vi "CRYTree Manuplate.vi"(4 "sData":string[](array[string]), 6 "Type":enum16{"Curves", "Values", "Results", "WFM"}(ring), 7 "sAction":string, 8 "sData Sub":string[](array[string]), 9 "nData":i32[](array[numeric]), 10 "sOption":string, 11 "Tree in":refnum<vi>) -> (0 "bResult Out":bool, 1 "sData Out":string[](array[string]), 2 "nData Out":i32[](array[numeric]), 3 "Tree Out":refnum<vi>)   [LabVIEW 2013]
uses:
  Global/CRYCurve Library Global.vi
panel:
  in  "Tags":string[](array[string])
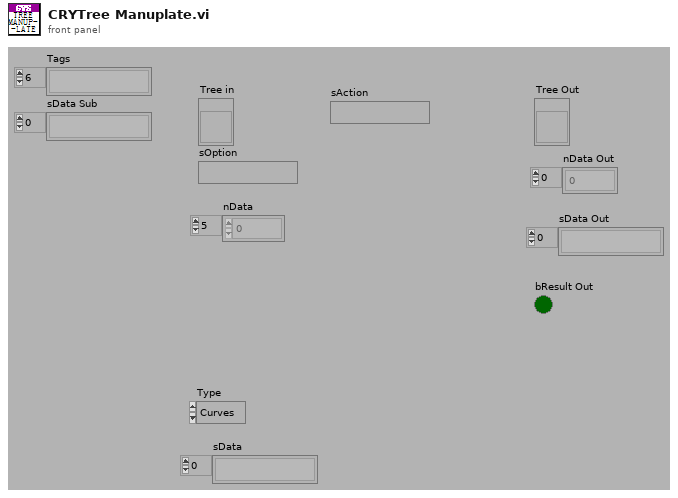
[diagram p1: front panel]
types:
  T1 = cluster{"Active Item Row Number":i32, "nData 2":i32}
  T2 = cluster{"Active Item Row Number":i32, "nData 2":i32}[]
  T3 = typedef "CRYCurveLib Info Cluster.ctl" = cluster{"GroupingState":string}
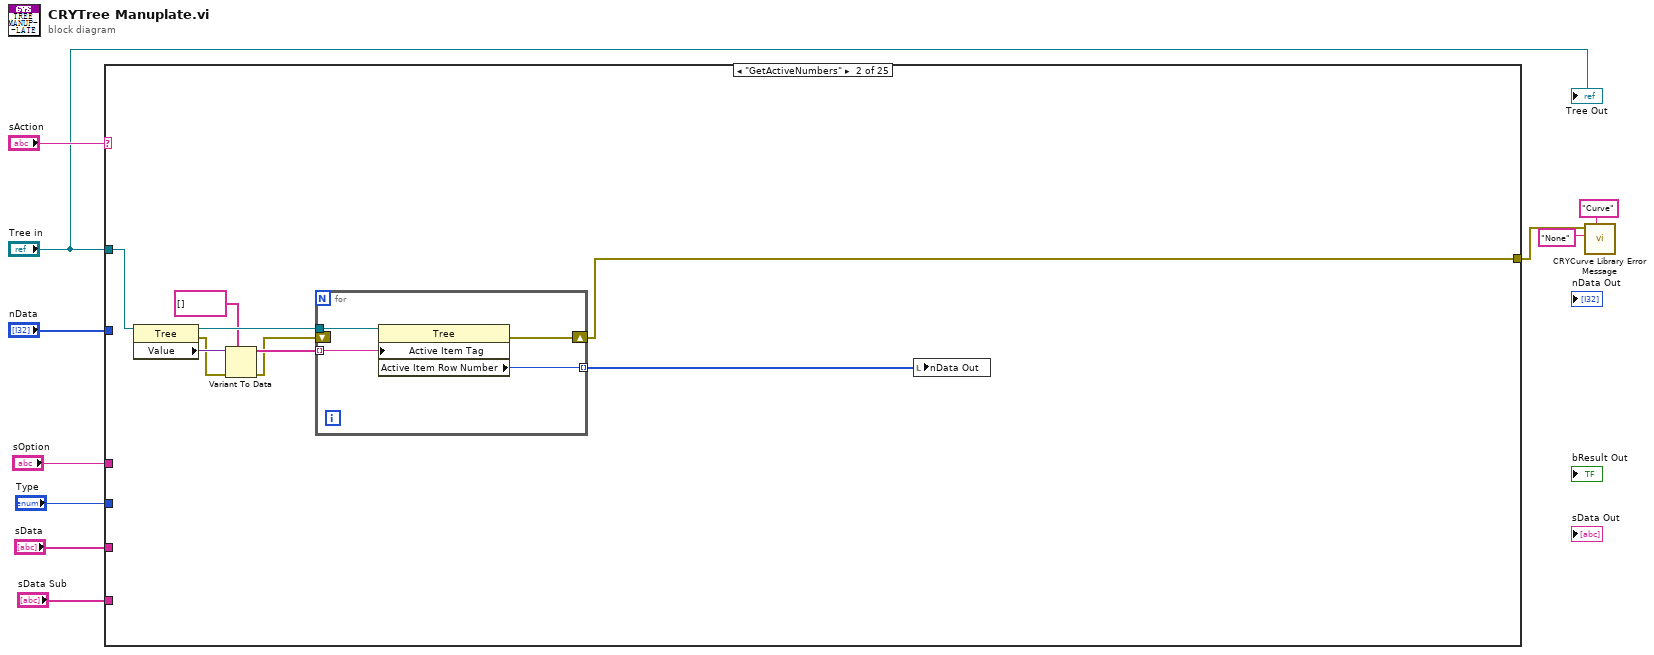
[diagram p0: block diagram]
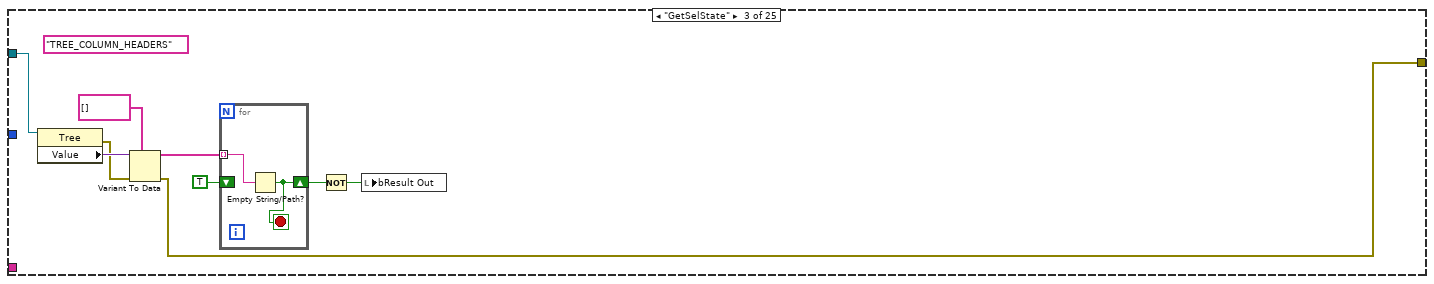
[diagram p3: hidden frame]
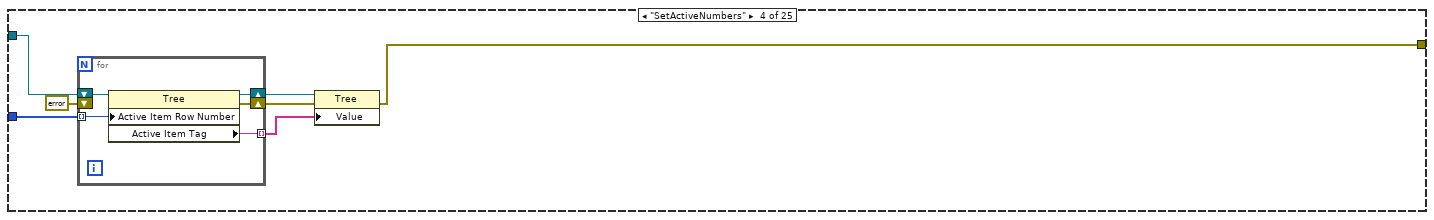
[diagram p4: hidden frame]
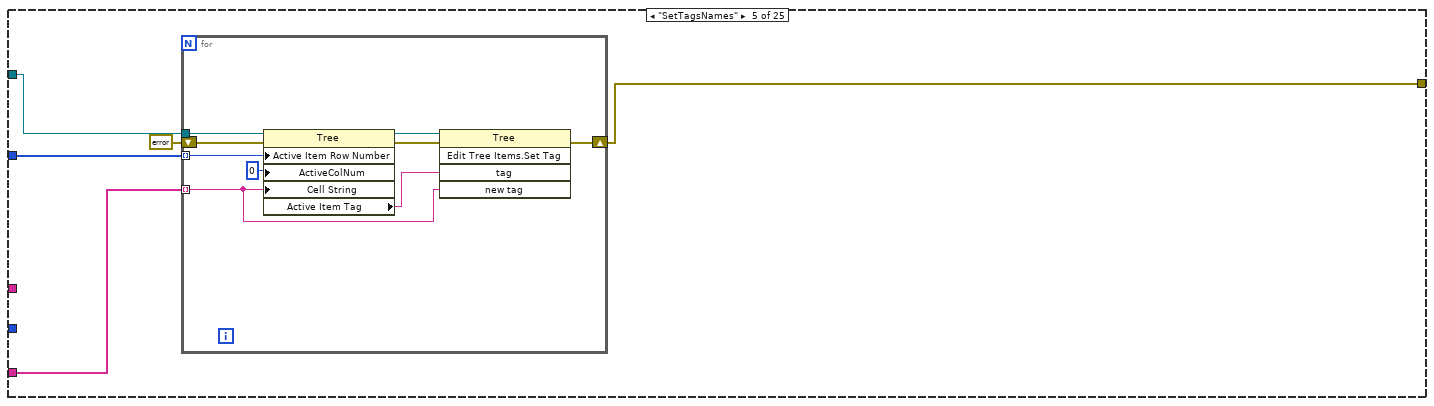
[diagram p5: hidden frame]
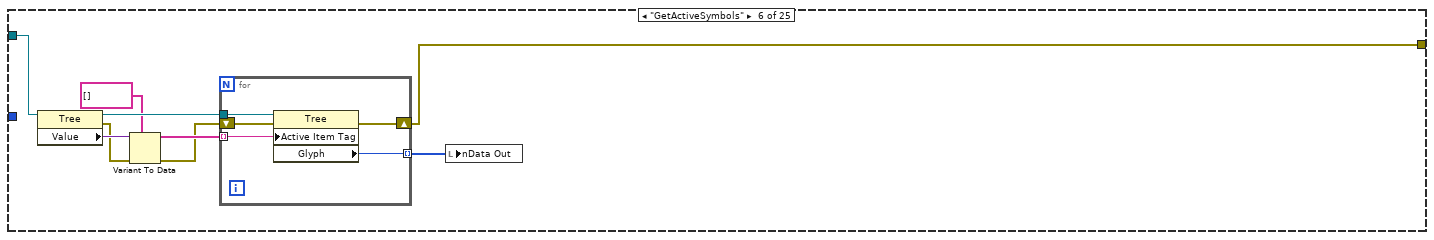
[diagram p6: hidden frame]
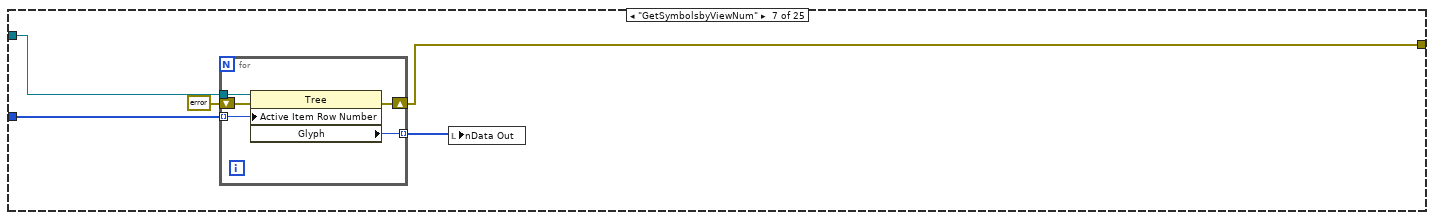
[diagram p7: hidden frame]
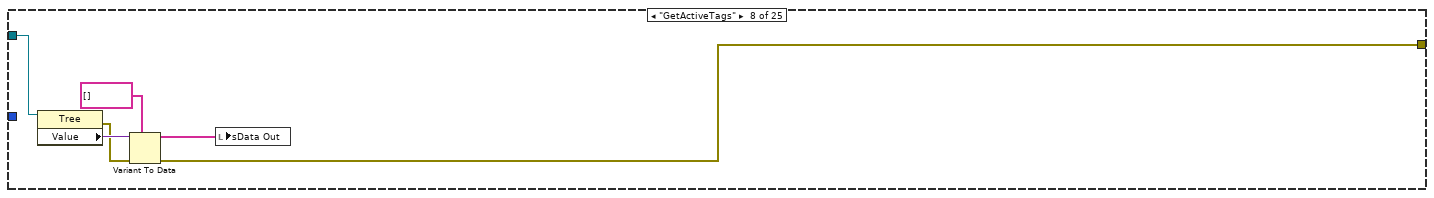
[diagram p8: hidden frame]
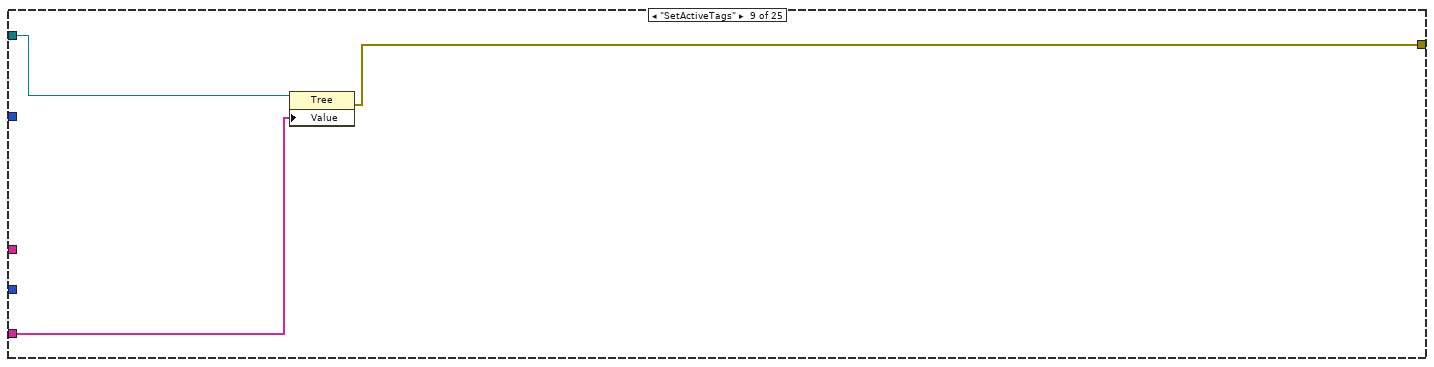
[diagram p9: hidden frame]
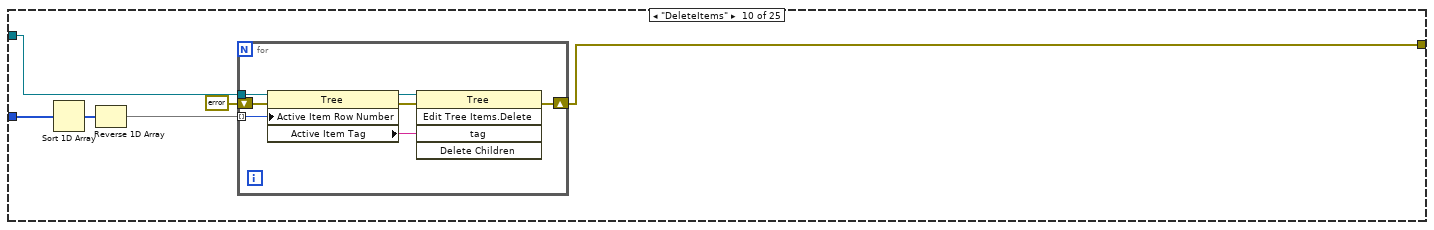
[diagram p10: hidden frame]
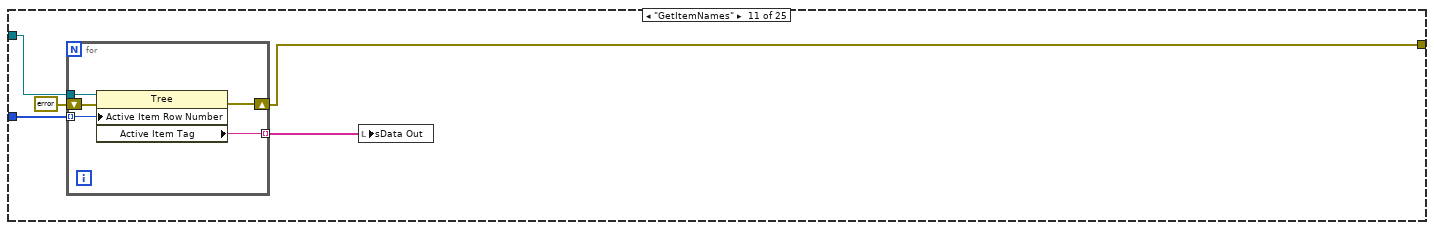
[diagram p11: hidden frame]
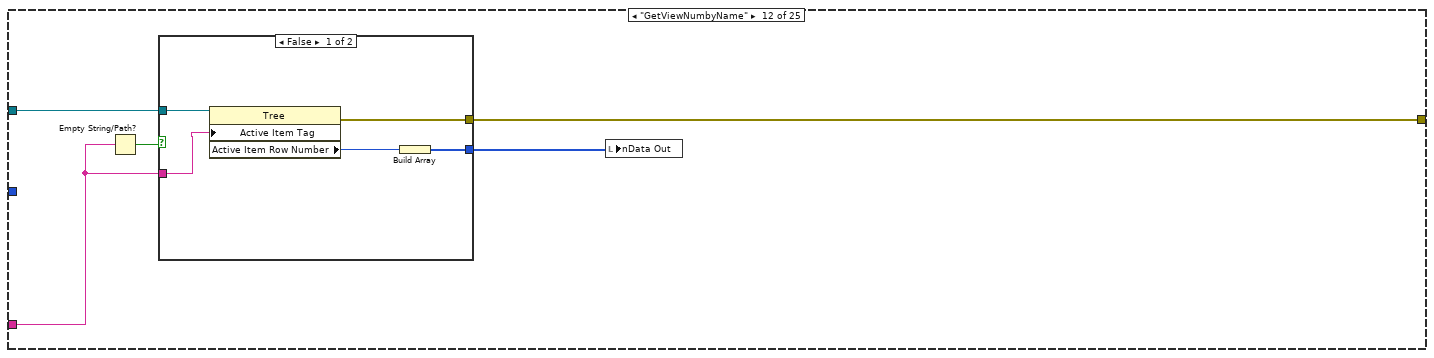
[diagram p12: hidden frame]
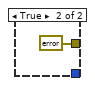
[diagram p13: hidden frame]
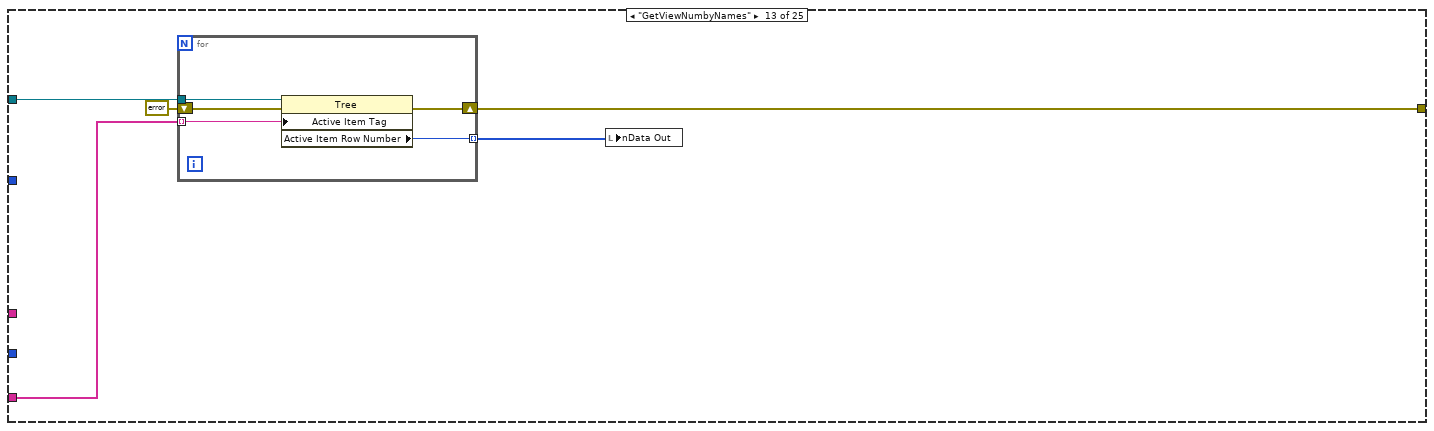
[diagram p14: hidden frame]
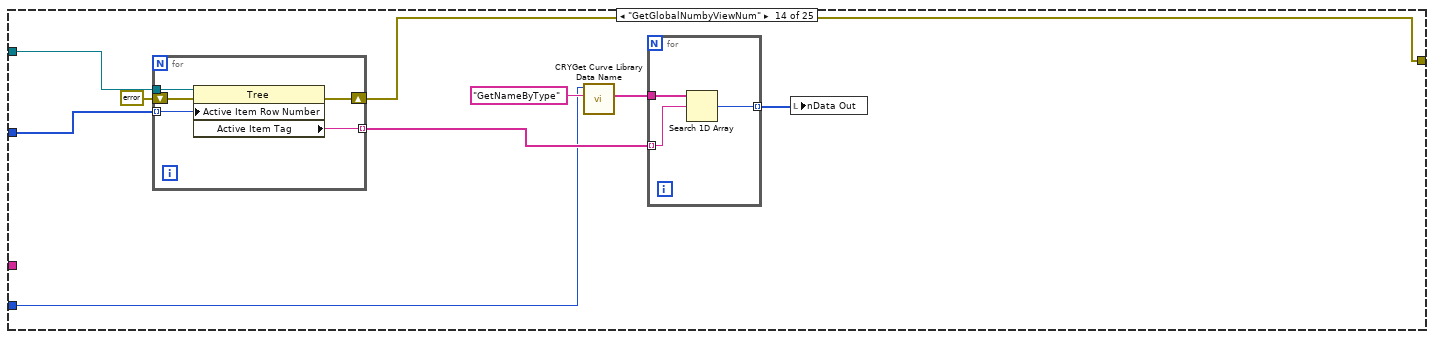
[diagram p15: hidden frame]
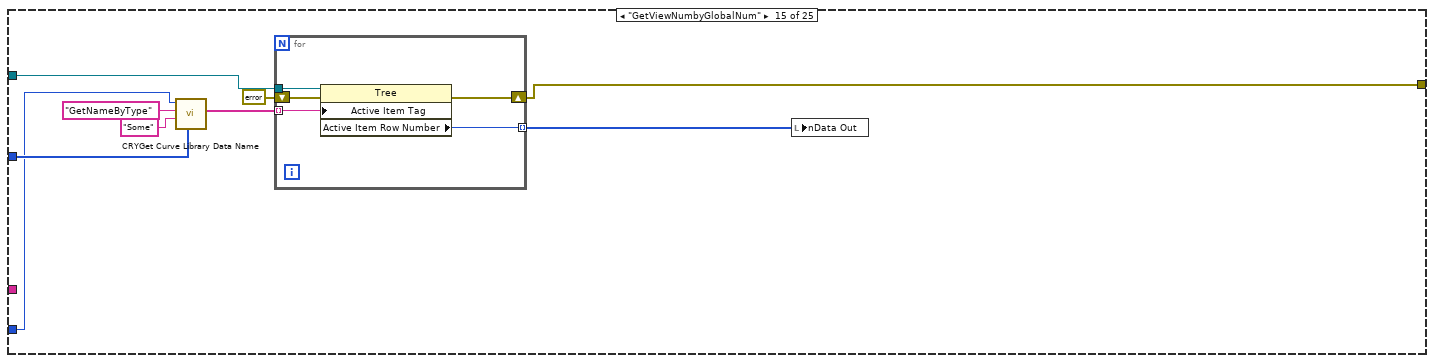
[diagram p16: hidden frame]
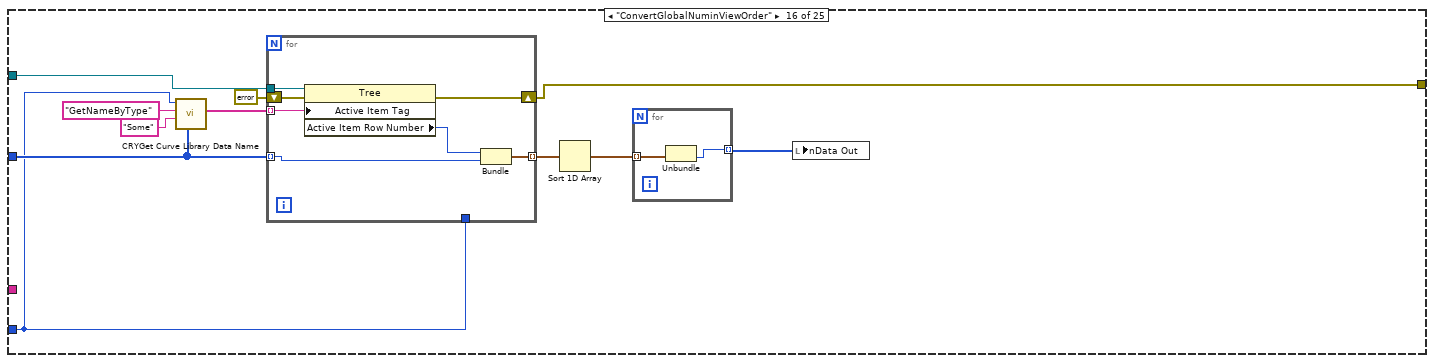
[diagram p17: hidden frame]
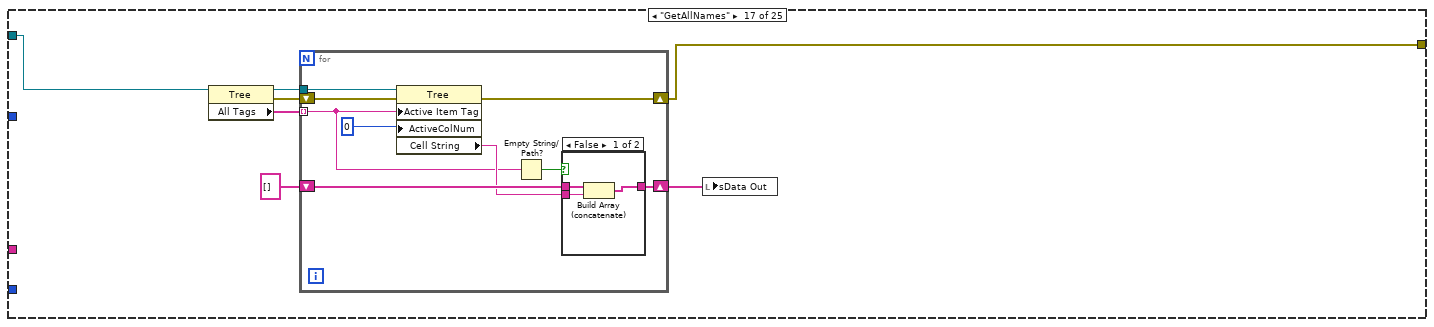
[diagram p18: hidden frame]
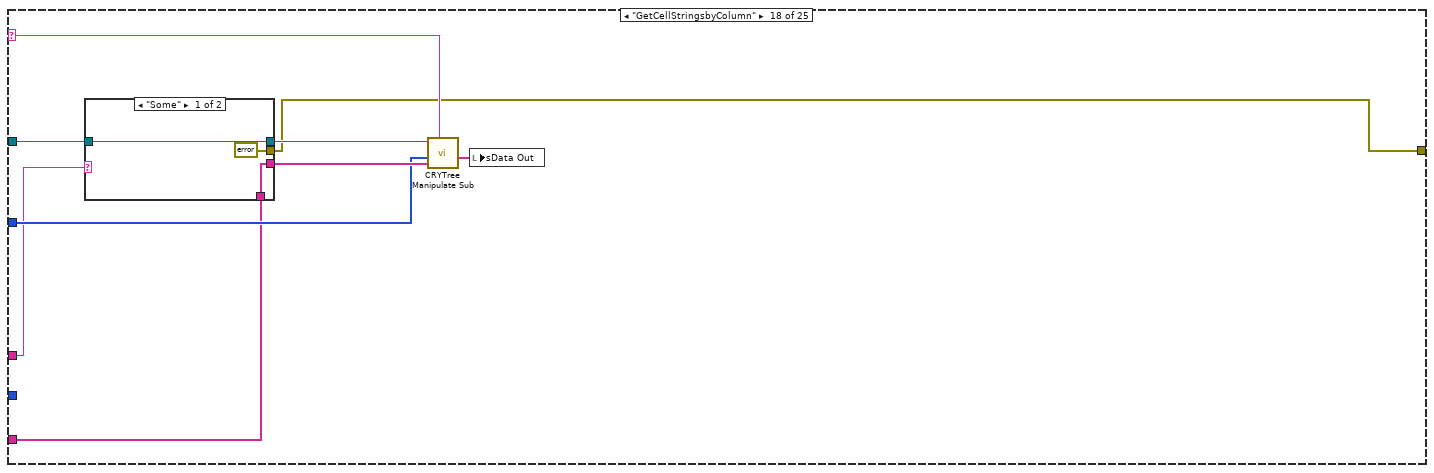
[diagram p20: hidden frame]
diagram:
  n1 = case shown="\"GetActiveNumbers\"" "sAction" {
    selector: "sAction" -> [_ _ _ _ _ _ _ _ _ _ _ _ _ _ _ _ _ w212 _ _ _ _ _ _ _]
    tunnel: "Tree in" -> [_ w16 w30 w41 w51 w65 w77 w88 w93 w99 w111 w121 w132 w146 w163 w176 w193 w214 w229 w245 w257 w327 w372 w735 w761]
    tunnel: "nData" -> [_ _ _ w39 w50 _ w78 _ _ w97 w110 _ _ w145 w160 w172 _ w216 _ _ w256 _ w373 w732 w763]
    tunnel: "sOption" -> [_ _ _ _ _ _ _ _ _ _ _ w118 _ _ _ _ _ w211 _ _ w252 _ w369 _ _]
    tunnel: "Type" -> [_ _ _ _ _ _ _ _ _ _ _ _ _ w140 w157 w171 _ _ _ _ _ _ _ _ _]
    tunnel: "sData" -> [_ _ _ _ w49 _ _ _ w92 _ _ _ w130 _ _ _ _ w210 _ _ _ w325 w368 _ w760]
    tunnel: "sData Sub" -> [_ _ _ _ _ _ _ _ _ _ _ _ _ _ _ _ _ _ _ _ _ _ _ _ _]
    tunnel: [_ w13 w24 w35 w48 w61 w75 w85 w91 w95 w108 w117 w128 w139 w156 w170 w189 w209 w226 w244 w251 w323 w367 w726 w759] -> w1
    frame Default {
    }
    frame "GetActiveNumbers" {
      n2 = property class="Tree"(reference=w16) -> (reference out=w17:refnum<vi>, error out=w12:errorcluster, "Value"=w19:variant)  [unwired: 1 in]
      n3 = Variant To Data(error in=w12, type=string[] [] ("Value"), Variant=w19) -> (data=w18:string[], error out=w11:errorcluster)
      n4 = for {
        tunnel: w17 -> [w23]
        tunnel: w18 -> [w21] mode=indexing
        tunnel: [w22] -> w15 mode=indexing
        shift-right: [w20] -> w13
        shift-left: w11 -> [_]
        n5 = property class="Tree"(reference=w23, "Active Item Tag"=w21) -> (error out=w20:errorcluster, "Active Item Row Number"=w22:i32)  [unwired: 1 in, 1 out]
      }
      n6 = local write "nData Out"(w15) -> ()
    }
    frame "GetSelState" {
      (unwired) "TREE_COLUMN_HEADERS" ("x")
      n7 = property class="Tree"(reference=w30) -> (error out=w25:errorcluster, "Value"=w32:variant)  [unwired: 1 in, 1 out]
      n8 = Variant To Data(error in=w25, type=string[] [] ("Value"), Variant=w32) -> (data=w31:string[], error out=w24:errorcluster)
      n9 = for {
        tunnel: w31 -> [w34] mode=indexing
        shift-right: [w33] -> w27
        shift-left: TRUE -> [_]
        stop <- w33 stop-if-true
        n10 = Empty String/Path?(string/path=w34) -> (empty?=w33:bool)
      }
      n11 = Not(x=w27) -> (.not. x?=w26:bool)
      n12 = local write "bResult Out"(w26) -> ()
    }
    frame "SetActiveNumbers" {
      n13 = for {
        tunnel: [w45] -> w38 mode=indexing
        tunnel: w39 -> [w43] mode=indexing
        shift-right: [w44] -> w40
        shift-left: w41 -> [w46]
        shift-right: [w42] -> w37
        shift-left: errorcluster {"status"=FALSE, "code"=0, "source"=""} ("error out") -> [_]
        n14 = property class="Tree"(reference=w46, "Active Item Row Number"=w43) -> (reference out=w44:refnum<vi>, error out=w42:errorcluster, "Active Item Tag"=w45:string)  [unwired: 1 in]
      }
      n15 = property class="Tree"(reference=w40, error in=w37, "Value"=w38) -> (error out=w35:errorcluster)  [unwired: 1 out]
    }
    frame "SetTagsNames" {
      n16 = for {
        tunnel: w50 -> [w60] mode=indexing
        tunnel: w51 -> [w58]
        tunnel: w49 -> [w56] mode=indexing
        shift-right: [w54] -> w48
        shift-left: errorcluster {"status"=FALSE, "code"=0, "source"=""} ("error out") -> [w53]
        n17 = property class="Tree"(reference=w58, error in=w53, "Active Item Row Number"=w60, "ActiveColNum"=0 ("Active Cell:Active Column Number"), "Cell String"=w56) -> (reference out=w57:refnum<vi>, error out=w52:errorcluster, "Active Item Tag"=w55:string)
        n18 = invoke class="Tree" method="Edit Tree Items.Set Tag"(reference=w57, error in=w52, "tag"=w55, "new tag"=w56) -> (error out=w54:errorcluster)  [unwired: 1 in, 4 out]
      }
    }
    frame "GetActiveSymbols" {
      n19 = property class="Tree"(reference=w65) -> (reference out=w67:refnum<vi>, error out=w63:errorcluster, "Value"=w69:variant)  [unwired: 1 in]
      n20 = Variant To Data(error in=w63, type=string[] [] ("Selected Rows"), Variant=w69) -> (data=w68:string[], error out=w62:errorcluster)
      n21 = for {
        tunnel: w67 -> [w74]
        tunnel: w68 -> [w72] mode=indexing
        tunnel: [w73] -> w64 mode=indexing
        shift-right: [w70] -> w61
        shift-left: w62 -> [w71]
        n22 = property class="Tree"(reference=w74, error in=w71, "Active Item Tag"=w72) -> (error out=w70:errorcluster, "Glyph"=w73:i32)  [unwired: 1 out]
      }
      n23 = local write "nData Out"(w64) -> ()
    }
    frame "GetSymbolsbyViewNum" {
      n24 = for {
        tunnel: w77 -> [w84]
        tunnel: w78 -> [w83] mode=indexing
        tunnel: [w82] -> w79 mode=indexing
        shift-right: [w81] -> w75
        shift-left: errorcluster {"status"=FALSE, "code"=0, "source"=""} ("error out") -> [w80]
        n25 = property class="Tree"(reference=w84, error in=w80, "Active Item Row Number"=w83) -> (error out=w81:errorcluster, "Glyph"=w82:i32)  [unwired: 1 out]
      }
      n26 = local write "nData Out"(w79) -> ()
    }
    frame "GetActiveTags" {
      n27 = property class="Tree"(reference=w88) -> (error out=w86:errorcluster, "Value"=w90:variant)  [unwired: 1 in, 1 out]
      n28 = Variant To Data(error in=w86, type=string[] [] ("Selected Rows"), Variant=w90) -> (data=w87:string[], error out=w85:errorcluster)
      n29 = local write "sData Out"(w87) -> ()
    }
    frame "SetActiveTags" {
      n30 = property class="Tree"(reference=w93, "Value"=w92) -> (error out=w91:errorcluster)  [unwired: 1 in, 1 out]
    }
    frame "DeleteItems" {
      n31 = Sort 1D Array(array=w97) -> (sorted array=w98:i32[])
      n32 = Reverse 1D Array(array=w98) -> (reversed array=w96:i32[])
      n33 = for {
        tunnel: w99 -> [w105]
        tunnel: w96 -> [w104] mode=indexing
        shift-right: [w101] -> w95
        shift-left: errorcluster {"status"=FALSE, "code"=0, "source"=""} ("error out") -> [w100]
        n34 = property on="Property Node" class="Tree"(reference=w105, error in=w100, "Active Item Row Number"=w104) -> (reference out=w103:refnum<vi>, error out=w102:errorcluster, "Active Item Tag"=w106:string)
        n35 = invoke class="Tree" method="Edit Tree Items.Delete"(reference=w103, error in=w102, "tag"=w106) -> (error out=w101:errorcluster)  [unwired: 2 in, 4 out]
      }
    }
    frame "GetItemNames" {
      n36 = for {
        tunnel: w111 -> [w116]
        tunnel: w110 -> [w115] mode=indexing
        tunnel: [w114] -> w109 mode=indexing
        shift-right: [w113] -> w108
        shift-left: errorcluster {"status"=FALSE, "code"=0, "source"=""} ("error out") -> [w112]
        n37 = property on="Property Node" class="Tree"(reference=w116, error in=w112, "Active Item Row Number"=w115) -> (error out=w113:errorcluster, "Active Item Tag"=w114:string)  [unwired: 1 out]
      }
      n38 = local write "sData Out"(w109) -> ()
    }
    frame "GetViewNumbyName" {
      n39 = Empty String/Path?(string/path=w118) -> (empty?=w119:bool)
      n40 = case shown="False" w119 {
        tunnel: w121 -> [w126 _]
        tunnel: [w124 _] -> w120
        tunnel: w118 -> [w123 _]
        tunnel: [w122 errorcluster {"status"=FALSE, "code"=0, "source"=""} ("error out")] -> w117
        frame False {
          n41 = property class="Tree"(reference=w126, "Active Item Tag"=w123) -> (error out=w122:errorcluster, "Active Item Row Number"=w125:i32)  [unwired: 1 in, 1 out]
          n42 = Build Array(w125) -> (w124:i32[])
        }
        frame True {
        }
      }
      n43 = local write "nData Out"(w120) -> ()
    }
    frame "GetViewNumbyNames" {
      n44 = for {
        tunnel: w132 -> [w137]
        tunnel: [w136] -> w131 mode=indexing
        tunnel: w130 -> [w135] mode=indexing
        shift-right: [w134] -> w128
        shift-left: errorcluster {"status"=FALSE, "code"=0, "source"=""} ("error out") -> [w133]
        n45 = property class="Tree"(reference=w137, error in=w133, "Active Item Tag"=w135) -> (error out=w134:errorcluster, "Active Item Row Number"=w136:i32)  [unwired: 1 out]
      }
      n46 = local write "nData Out"(w131) -> ()
    }
    frame "GetGlobalNumbyViewNum" {
      n47 = for {
        tunnel: w146 -> [w154]
        tunnel: w145 -> [w153] mode=indexing
        tunnel: [w152] -> w143 mode=indexing
        shift-right: [w151] -> w139
        shift-left: errorcluster {"status"=FALSE, "code"=0, "source"=""} ("error out") -> [w150]
        n48 = property on="Property Node" class="Tree"(reference=w154, error in=w150, "Active Item Row Number"=w153) -> (error out=w151:errorcluster, "Active Item Tag"=w152:string)  [unwired: 1 out]
      }
      n49 = call "CRYGet Curve Library Data Name.vi"("sAction"="GetNameByType", "Type"=w140) -> ("sNames"=w142:string[])  [unwired: 6 in, 3 out]
      n50 = for {
        tunnel: w143 -> [w148] mode=indexing
        tunnel: w142 -> [w149]
        tunnel: [w147] -> w141 mode=indexing
        n51 = Search 1D Array(1D array=w149, element=w148) -> (index of element=w147:i32)  [unwired: 1 in]
      }
      n52 = local write "nData Out"(w141) -> ()
    }
    frame "GetViewNumbyGlobalNum" {
      n53 = call "CRYGet Curve Library Data Name.vi"("nData"=w160, "sOption"="Some", "sAction"="GetNameByType", "Type"=w157) -> ("sNames"=w159:string[])  [unwired: 4 in, 3 out]
      n54 = for {
        tunnel: w163 -> [w168]
        tunnel: w159 -> [w166] mode=indexing
        tunnel: [w167] -> w158 mode=indexing
        shift-right: [w165] -> w156
        shift-left: errorcluster {"status"=FALSE, "code"=0, "source"=""} ("error out") -> [w164]
        n55 = property on="Property Node" class="Tree"(reference=w168, error in=w164, "Active Item Tag"=w166) -> (error out=w165:errorcluster, "Active Item Row Number"=w167:i32)  [unwired: 1 out]
      }
      n56 = local write "nData Out"(w158) -> ()
    }
    frame "ConvertGlobalNuminViewOrder" {
      n57 = call "CRYGet Curve Library Data Name.vi"("nData"=w172, "sOption"="Some", "sAction"="GetNameByType", "Type"=w171) -> ("sNames"=w177:string[])  [unwired: 4 in, 3 out]
      n58 = for {
        tunnel: w176 -> [w188]
        tunnel: w177 -> [w184] mode=indexing
        tunnel: [w186] -> w175 mode=indexing
        tunnel: w172 -> [w185] mode=indexing
        tunnel: w171 -> [_]
        shift-right: [w183] -> w170
        shift-left: errorcluster {"status"=FALSE, "code"=0, "source"=""} ("error out") -> [w182]
        n59 = property on="Property Node" class="Tree"(reference=w188, error in=w182, "Active Item Tag"=w184) -> (error out=w183:errorcluster, "Active Item Row Number"=w187:i32)  [unwired: 1 out]
        n60 = Bundle("Active Item Row Number"=w187, "nData 2"=w185) -> (w186:T1)  [unwired: 1 in]
      }
      n61 = Sort 1D Array(array=w175) -> (sorted array=w174:T2)
      n62 = for {
        tunnel: w174 -> [w181] mode=indexing
        tunnel: [w180] -> w173 mode=indexing
        n63 = Unbundle(w181) -> ("nData 2"=w180:i32)  [unwired: 1 out]
      }
      n64 = local write "nData Out"(w173) -> ()
    }
    frame "GetAllNames" {
      n65 = property class="Tree"(reference=w193) -> (reference out=w192:refnum<vi>, error out=w190:errorcluster, "All Tags"=w191:string[])  [unwired: 1 in]
      n66 = for {
        tunnel: w192 -> [w199]
        shift-right: [w202] -> w195
        shift-left: string[] [] -> [w203]
        tunnel: w191 -> [w198] mode=indexing
        shift-right: [w196] -> w189
        shift-left: w190 -> [w197]
        n67 = property class="Tree"(reference=w199, error in=w197, "Active Item Tag"=w198, "ActiveColNum"=0 ("Active Cell:Active Column Number")) -> (error out=w196:errorcluster, "Cell String"=w200:string)  [unwired: 1 out]
        n68 = Empty String/Path?(string/path=w198) -> (empty?=w204:bool)
        n69 = case shown="False" w204 {
          tunnel: w203 -> [w207 w208]
          tunnel: w200 -> [w206 _]
          tunnel: [w205 w208] -> w202
          frame False {
            n70 = Build Array (concatenate)(w207, w206) -> (w205:string[])
          }
          frame True {
          }
        }
      }
      n71 = local write "sData Out"(w195) -> ()
    }
    frame "GetCellStringsbyColumn" {
      n72 = case shown="\"Some\"" w211 {
        tunnel: [w219 w224] -> w217
        tunnel: w214 -> [w220 w223]
        tunnel: [w220 w222] -> w213
        tunnel: w210 -> [w219 _]
        tunnel: [errorcluster {"status"=FALSE, "code"=0, "source"=""} ("error out") w221] -> w209
        frame "Some" {
        }
        frame Default {
          n73 = property class="Tree"(reference=w223) -> (reference out=w222:refnum<vi>, error out=w221:errorcluster, "All Tags"=w224:string[])  [unwired: 1 in]
        }
      }
      n74 = call "CRYTree Manipulate Sub.vi"("sAction"=w212, "sData"=w217, "nData"=w216, "Tree in"=w213) -> ("sData Out"=w215:string[])  [unwired: 3 in, 4 out]
      n75 = local write "sData Out"(w215) -> ()
    }
    frame "GetItemSymbols" {
      n76 = property class="Tree"(reference=w229) -> (reference out=w228:refnum<vi>, error out=w225:errorcluster, "All Tags"=w227:string[])  [unwired: 1 in]
      n77 = for {
        tunnel: w228 -> [w233]
        shift-right: [w238] -> w226
        shift-left: w225 -> [w234]
        shift-right: [w236] -> w231
        shift-left: i32[] [] -> [w235]
        tunnel: w227 -> [w232] mode=indexing
        n78 = property class="Tree"(reference=w233, error in=w234, "Active Item Tag"=w232) -> (error out=w238:errorcluster, "Glyph"=w237:i32)  [unwired: 1 out]
        n79 = Empty String/Path?(string/path=w232) -> (empty?=w239:bool)
        n80 = case shown="False" w239 {
          tunnel: w237 -> [w242 _]
          tunnel: [w241 w243] -> w236
          tunnel: w235 -> [w240 w243]
          frame False {
            n81 = Build Array (concatenate)(w240, w242) -> (w241:i32[])
          }
          frame True {
          }
        }
      }
      n82 = local write "nData Out"(w231) -> ()
    }
    frame "GetTotalCount" {
      n83 = property class="Tree"(reference=w245) -> (error out=w244:errorcluster, "All Tags"=w246:string[])  [unwired: 1 in, 1 out]
      n84 = Array Size(array=w246) -> (size(s)=w247:i32)
      n85 = Build Array(w247) -> (w248:i32[])
      n86 = local write "nData Out"(w248) -> ()
    }
    frame "GetAllChild" {
      n87 = for {
        tunnel: w256 -> [w277] mode=indexing
        tunnel: w257 -> [w278]
        shift-right: [w274] -> w255
        shift-left: string[] [] ("Tags") -> [w275]
        tunnel: w252 -> [w267]
        shift-right: [w263] -> w250
        shift-left: errorcluster {"status"=FALSE, "code"=0, "source"=""} ("error out") -> [w266]
        n88 = flat-sequence {
          tunnel: w275 -> [w283]
          tunnel: w277 -> [w284]
          tunnel: w278 -> [w285]
          tunnel: [w285] -> w272
          tunnel: [w284] -> w271
          tunnel: [w283] -> w270
          tunnel: [w281] -> w268
          tunnel: w267 -> [w281]
          tunnel: w266 -> [w280]
          tunnel: [w279] -> w265
          tunnel: [w290] -> w276
          tunnel: [w289] -> w273
          tunnel: w272 -> [w294]
          tunnel: w271 -> [w291]
          tunnel: w270 -> [w290]
          tunnel: [w288] -> w269
          tunnel: w268 -> [w288]
          tunnel: w265 -> [w287]
          tunnel: [w286] -> w264
          tunnel: w276 -> [w302]
          tunnel: [w301] -> w274
          tunnel: w273 -> [w300]
          tunnel: w269 -> [w299]
          tunnel: w264 -> [w297]
          tunnel: [w296] -> w263
          frame #0 {
            n89 = property on="Tags" class="Arr (strict)"(error in=w280, "Value"=string[] [] ("Tags")) -> (error out=w279:errorcluster)  [unwired: 1 in, 1 out]
          }
          frame #1 {
            n90 = property class="Tree"(reference=w294, error in=w287, "Active Item Row Number"=w291) -> (reference out=w293:refnum<vi>, error out=w286:errorcluster, "Active Item Tag"=w292:string)
            n91 = control-ref of="Tags"() -> (w295:refnum<vi>)
            n92 = call "CRYTree Navigate.vi"("Tags"=w295, "Start Tag In"=w292, "Tree In"=w293) -> ("Tree Out"=w289:refnum<vi>)  [unwired: 8 in]
          }
          frame #2 {
            n93 = property on="Tags" class="Arr (strict)"(error in=w297) -> (error out=w296:errorcluster, "Value"=w298:string[])  [unwired: 1 in, 1 out]
            n94 = case shown="Default" w299 {
              tunnel: w302 -> [w304 w309]
              tunnel: [w303 w308] -> w301
              tunnel: w300 -> [_ w307]
              tunnel: w298 -> [w305 w306]
              frame "WithGroup" {
                n95 = Insert Into Array(array=w304, new element=w305) -> (w303:string[])  [unwired: 1 in]
              }
              frame Default {
                n96 = for {
                  tunnel: w307 -> [w312]
                  shift-right: [w316] -> w308
                  shift-left: w309 -> [w317]
                  tunnel: w306 -> [w310] mode=indexing
                  n97 = Build Array(w310) -> (w315:string[])
                  n98 = call "CRYTree Manipulate Sub.vi"("sAction"="CheckGroup", "sData"=w315, "sOption"="byTag", "Tree in"=w312) -> ("bData out"=w311:bool)  [unwired: 3 in, 4 out]
                  n99 = case shown="False" w311 {
                    tunnel: w317 -> [w320 w321]
                    tunnel: [w319 w321] -> w316
                    tunnel: w310 -> [w318 _]
                    frame False {
                      n100 = Insert Into Array(array=w320, new element=w318) -> (w319:string[])  [unwired: 1 in]
                    }
                    frame True {
                    }
                  }
                }
              }
            }
          }
        }
      }
      n101 = for {
        tunnel: w257 -> [w262]
        tunnel: w255 -> [w261] mode=indexing
        tunnel: [w260] -> w253 mode=indexing
        shift-right: [w259] -> w251
        shift-left: w250 -> [w258]
        n102 = property class="Tree"(reference=w262, error in=w258, "Active Item Tag"=w261) -> (error out=w259:errorcluster, "Active Item Row Number"=w260:i32)  [unwired: 1 out]
      }
      n103 = local write "sData Out"(w255) -> ()
      n104 = local write "nData Out"(w253) -> ()
    }
    frame "GetAllParents" {
      n105 = for {
        tunnel: w325 -> [w333] mode=indexing
        shift-right: [w330] -> w324
        shift-left: string[] [] ("sData") -> [w331]
        n106 = Empty String/Path?(string/path=w333) -> (empty?=w334:bool)
        n107 = Build Array (concatenate)(w331, w333) -> (w332:string[])
        n108 = Select(t=w331, s=w334, f=w332) -> (s? t:f=w330:string[])
      }
      n109 = for {
        tunnel: w324 -> [w338] mode=indexing
        tunnel: w327 -> [w340]
        shift-right: [w345] -> w328
        shift-left: string[] [] ("sData") -> [w344]
        shift-right: [w336] -> w323
        shift-left: errorcluster {"status"=FALSE, "code"=0, "source"=""} ("error out") -> [w335]
        n110 = Build Array(w338) -> (w337:string[])
        n111 = call "CRYTree Manipulate Sub.vi"("sAction"="CheckGroup", "sData"=w337, "sOption"="byTag", "Tree in"=w340) -> ("bData out"=w339:bool)  [unwired: 3 in, 4 out]
        n112 = case shown="True" w339 {
          tunnel: w344 -> [w346 w349]
          tunnel: [w346 w348] -> w343
          tunnel: w338 -> [_ w347]
          frame False {
          }
          frame True {
            n113 = Insert Into Array(array=w349, new element=w347) -> (w348:string[])  [unwired: 1 in]
          }
        }
        n114 = while {
          tunnel: w340 -> [w361]
          shift-right: [w359] -> w345
          shift-left: w343 -> [w358]
          shift-right: [w352] -> _
          shift-left: w338 -> [w360]
          shift-right: [w351] -> w336
          shift-left: w335 -> [w350]
          stop <- w355 stop-if-true
          n115 = invoke class="Tree" method="Navigate Tree.Get Parent"(reference=w361, error in=w350, "tag"=w360) -> (error out=w351:errorcluster, "Navigate Tree:Get Parent"=w357:string)  [unwired: 1 in, 2 out]
          n116 = Empty String/Path?(string/path=w357) -> (empty?=w356:bool)
          n117 = Search 1D Array(1D array=w358, element=w357) -> (index of element=w354:i32)  [unwired: 1 in]
          n118 = Greater Or Equal To 0?(x=w354) -> (x >= 0?=w353:bool)
          n119 = Compound Arithmetic op=OR(w356, w353) -> (w355:bool)
          n120 = case shown="False" w355 {
            tunnel: w357 -> [w362 w365]
            tunnel: w358 -> [w364 w366]
            tunnel: [w363 w366] -> w359
            tunnel: [w362 w365] -> w352
            frame False {
              n121 = Insert Into Array(array=w364, new element=w362) -> (w363:string[])  [unwired: 1 in]
            }
            frame True {
            }
          }
        }
      }
      n122 = local write "sData Out"(w328) -> ()
    }
    frame "FindInsertLoc" {
      n123 = case shown="\"Group\"" w369 {
        tunnel: w373 -> [w382 _ w436 w485 _ _ _ w589 w668 w716]
        tunnel: [w391 w420 w439 w494 w533 w554 w578 w590 w669 w711] -> w370
        tunnel: [w392 w421 w440 w495 w534 w555 w579 w591 _ w712] -> w371
        tunnel: w372 -> [w381 w414 w437 w484 w515 w535 w560 w583 w663 w713]
        tunnel: w368 -> [_ _ w438 _ w522 w543 w559 _ _ _]
        tunnel: [w376 _ w430 w478 w513 _ _ w580 w662 w705] -> w367
        frame "Group" {
          n124 = for {
            tunnel: w382 -> [w399] mode=indexing
            tunnel: w381 -> [w401]
            tunnel: [w398] -> w380 mode=indexing
            shift-right: [w397] -> w375
            shift-left: errorcluster {"status"=FALSE, "code"=0, "source"=""} ("error out") -> [w396]
            n125 = property on="Property Node" class="Tree"(reference=w401, error in=w396, "Active Item Row Number"=w399) -> (error out=w397:errorcluster, "Indent Level"=w400:i32)  [unwired: 1 out]
            n126 = Bundle("Indent Level"=w400, "nData 2"=w399) -> (w398:cluster{"Indent Level":i32, "nData 2":i32})  [unwired: 1 in]
          }
          n127 = Sort 1D Array(array=w380) -> (sorted array=w379:cluster{"Indent Level":i32, "nData 2":i32}[])
          n128 = Index Array(array=w379) -> (element=w378:cluster{"Indent Level":i32, "nData 2":i32})  [unwired: 1 in]
          n129 = Unbundle(w378) -> ("nData 2"=w377:i32)  [unwired: 1 out]
          n130 = property on="Property Node" class="Tree"(reference=w381, error in=w375, "Active Item Row Number"=w377) -> (reference out=w395:refnum<vi>, error out=w394:errorcluster, "Active Item Tag"=w393:string)
          n131 = invoke class="Tree" method="Navigate Tree.Get Parent"(reference=w395, error in=w394, "tag"=w393) -> (reference out=w388:refnum<vi>, error out=w376:errorcluster, "Navigate Tree:Get Parent"=w387:string)  [unwired: 1 in, 1 out]
          n132 = Build Array(w387) -> (w389:string[])
          n133 = call "CRYTree Manipulate Sub.vi"("sAction"="GetTags", "sData"=w389, "sOption"="Childs", "Tree in"=w388) -> ("sData Out"=w386:string[], "Tree Out"=w384:refnum<vi>)  [unwired: 3 in, 3 out]
          n134 = for {
            tunnel: w386 -> [w403] mode=indexing
            tunnel: [w406] -> w385
            tunnel: w384 -> [w404]
            i -> [w406]
            stop <- w407 stop-if-true
            n135 = Build Array(w403) -> (w402:string[])
            n136 = call "CRYTree Manipulate Sub.vi"("sAction"="CheckGroup", "sData"=w402, "sOption"="byTag", "Tree in"=w404) -> ("bData out"=w408:bool)  [unwired: 3 in, 4 out]
            n137 = Not(x=w408) -> (.not. x?=w407:bool)
          }
          n138 = Build Array(w387) -> (w392:string[])
          n139 = Build Array(w385) -> (w391:i32[])
        }
        frame "Grouping" {
          # "CRYGroup Manipulate.vi\\\"GroupingbyCategory\", \"GroupingbyStep\""
          n140 = Build Array("") -> (w418:string[])
          n141 = call "CRYTree Manipulate Sub.vi"("sAction"="GetTags", "sData"=w418, "sOption"="Childs", "Tree in"=w414) -> ("sData Out"=w412:string[], "Tree Out"=w417:refnum<vi>)  [unwired: 3 in, 3 out]
          n142 = for {
            tunnel: w412 -> [w424] mode=indexing
            tunnel: [w428] -> w411
            tunnel: w417 -> [w426]
            tunnel: [w424] -> w413
            tunnel: [w423] -> w410
            i -> [w428]
            stop <- w423 stop-if-true
            # "Only Group"
            n143 = Build Array(w424) -> (w425:string[])
            n144 = call "CRYTree Manipulate Sub.vi"("sAction"="CheckGroup", "sData"=w425, "sOption"="byTag", "Tree in"=w426) -> ("bOnlyGroup"=w422:bool)  [unwired: 3 in, 4 out]
            n145 = Not(x=w422) -> (.not. x?=w423:bool)
          }
          n146 = Build Array(w413) -> (w421:string[])
          n147 = Build Array(w411) -> (w420:i32[])
          n148 = local write "bResult Out"(w410) -> ()
        }
        frame "MovebyReplace" {
          # "CRYInsert Data to Listbox.vi"
          n149 = Index Array(array=w438) -> (element=w432:string)  [unwired: 1 in]
          n150 = Empty String/Path?(string/path=w432) -> (empty?=w433:bool)
          n151 = case shown="False" w433 {
            selector: w433 -> [_ w477]
            tunnel: w437 -> [w451 _]
            tunnel: w436 -> [w450 _]
            tunnel: [w449 _] -> w435
            tunnel: [w448 _] -> w434
            tunnel: w432 -> [w445 _]
            tunnel: [w442 w477] -> w431
            tunnel: [w441 _] -> w430
            frame False {
              n152 = invoke class="Tree" method="Navigate Tree.Get Parent"(reference=w451, "tag"=w445) -> (reference out=w446:refnum<vi>, error out=w441:errorcluster, "Navigate Tree:Get Parent"=w444:string)  [unwired: 2 in, 1 out]
              n153 = Empty String/Path?(string/path=w444) -> (empty?=w443:bool)
              n154 = case shown="False" w443 {
                tunnel: [w454 FALSE ("bData out")] -> w447
                tunnel: w446 -> [w453 _]
                tunnel: w444 -> [w452 _]
                frame False {
                  n155 = Build Array(w452) -> (w457:string[])
                  n156 = call "CRYTree Manipulate Sub.vi"("sAction"="CheckGroup", "sData"=w457, "sOption"="byTag", "Tree in"=w453) -> ("bData out"=w454:bool)  [unwired: 3 in, 4 out]
                }
                frame True {
                  # "Root is not Group."
                }
              }
              n157 = case shown="False" w447 {
                selector: w447 -> [_ w476]
                tunnel: w446 -> [w467 _]
                tunnel: w450 -> [w472 _]
                tunnel: [w461 _] -> w449
                tunnel: [w462 _] -> w448
                tunnel: w445 -> [w466 _]
                tunnel: w444 -> [w460 _]
                tunnel: [w459 w476] -> w442
                frame False {
                  n158 = Index Array(array=w472) -> (element #1=w475:i32, element #2=w474:i32)  [unwired: 2 in]
                  n159 = Build Array(w460) -> (w469:string[])
                  n160 = call "CRYTree Manipulate Sub.vi"("sAction"="GetTags", "sData"=w469, "sOption"="Childs", "Tree in"=w467) -> ("sData Out"=w471:string[])  [unwired: 3 in, 4 out]
                  n161 = call "CRYFind Insert Locaction in Tree.vi"("Index in Step"=w474, "Index in Tree"=w475, "ParentTag In"="", "Tree in"=w467) -> ("ChildIndex"=w462:i32, "ParentTag Out"=w461:string)  [unwired: 5 in, 1 out]
                  n162 = Search 1D Array(1D array=w471, element=w466) -> (index of element=w463:i32)  [unwired: 1 in]
                  n163 = Equal?(x=w460, y=w461) -> (x = y?=w465:bool)
                  n164 = Equal?(x=w463, y=w462) -> (x = y?=w464:bool)
                  n165 = And(x=w465, y=w464) -> (x .and. y?=w459:bool)
                }
                frame True {
                }
              }
            }
            frame True {
            }
          }
          n166 = local write "bResult Out"(w431) -> ()
          n167 = Build Array(w435) -> (w440:string[])
          n168 = Build Array(w434) -> (w439:i32[])
        }
        frame "Delete" {
          n169 = for {
            tunnel: w485 -> [w502] mode=indexing
            tunnel: w484 -> [w504]
            tunnel: [w501] -> w483 mode=indexing
            shift-right: [w500] -> w479
            shift-left: _ -> [w499]
            n170 = property on="Property Node" class="Tree"(reference=w504, error in=w499, "Active Item Row Number"=w502) -> (error out=w500:errorcluster, "Indent Level"=w503:i32)  [unwired: 1 out]
            n171 = Bundle("Indent Level"=w503, "nData 2"=w502) -> (w501:cluster{"Indent Level":i32, "nData 2":i32})  [unwired: 1 in]
          }
          n172 = Sort 1D Array(array=w483) -> (sorted array=w482:cluster{"Indent Level":i32, "nData 2":i32}[])
          n173 = Index Array(array=w482) -> (element=w481:cluster{"Indent Level":i32, "nData 2":i32})  [unwired: 1 in]
          n174 = Unbundle(w481) -> ("nData 2"=w480:i32)  [unwired: 1 out]
          n175 = property on="Property Node" class="Tree"(reference=w484, error in=w479, "Active Item Row Number"=w480) -> (reference out=w498:refnum<vi>, error out=w497:errorcluster, "Active Item Tag"=w496:string)
          n176 = invoke class="Tree" method="Navigate Tree.Get Parent"(reference=w498, error in=w497, "tag"=w496) -> (reference out=w491:refnum<vi>, error out=w478:errorcluster, "Navigate Tree:Get Parent"=w490:string)  [unwired: 1 in, 1 out]
          n177 = Build Array(w490) -> (w492:string[])
          n178 = call "CRYTree Manipulate Sub.vi"("sAction"="GetTags", "sData"=w492, "sOption"="Childs", "Tree in"=w491) -> ("sData Out"=w489:string[], "Tree Out"=w487:refnum<vi>)  [unwired: 3 in, 3 out]
          n179 = for {
            tunnel: w489 -> [w506] mode=indexing
            tunnel: [w509] -> w488
            tunnel: w487 -> [w507]
            i -> [w509]
            stop <- w510 stop-if-true
            n180 = Build Array(w506) -> (w505:string[])
            n181 = call "CRYTree Manipulate Sub.vi"("sAction"="CheckGroup", "sData"=w505, "sOption"="byTag", "Tree in"=w507) -> ("bData out"=w511:bool)  [unwired: 3 in, 4 out]
            n182 = Not(x=w511) -> (.not. x?=w510:bool)
          }
          n183 = Build Array(w490) -> (w495:string[])
          n184 = Build Array(w488) -> (w494:i32[])
        }
        frame "Data" {
          # "Step Move Up and Down"
          n185 = Index Array(array=w522) -> (element=w521:string)  [unwired: 1 in]
          n186 = invoke class="Tree" method="Navigate Tree.Get Parent"(reference=w515, "tag"=w521) -> (reference out=w514:refnum<vi>, error out=w513:errorcluster, "Navigate Tree:Get Parent"=w520:string)  [unwired: 2 in, 1 out]
          n187 = Build Array(4 ("nData 2")) -> (w532:i32[])
          n188 = Build Array(5 ("nData 2")) -> (w527:i32[])
          n189 = call "CRYTree Manipulate Sub.vi"("sAction"="GetCellStringsbyColumn", "sData"=w522, "nData"=w532, "Tree in"=w514) -> ("sData Out"=w526:string[])  [unwired: 3 in, 4 out]
          n190 = call "CRYTree Manipulate Sub.vi"("sAction"="GetCellStringsbyColumn", "sData"=w522, "nData"=w527, "Tree in"=w514) -> ("sData Out"=w523:string[])  [unwired: 3 in, 4 out]
          n191 = Index Array(array=w526) -> (element=w525:string)  [unwired: 1 in]
          n192 = Index Array(array=w523) -> (element=w524:string)  [unwired: 1 in]
          n193 = Decimal String To Number(string=w525) -> (number=w517:i32)  [unwired: 2 in, 1 out]
          n194 = Decimal String To Number(string=w524) -> (number=w516:i32)  [unwired: 2 in, 1 out]
          n195 = call "CRYFind Insert Locaction in Tree.vi"("Index in Step"=w516, "Index in Tree"=w517, "ParentTag In"=w520, "Tree in"=w514) -> ("ChildIndex"=w518:i32, "ParentTag Out"=w519:string)  [unwired: 5 in, 1 out]
          n196 = Build Array(w519) -> (w534:string[])
          n197 = Build Array(w518) -> (w533:i32[])
        }
        frame "GroupData" {
          # "Grouping off"
          # "NewGroup, UnGroup"
          n198 = Index Array(array=w543) -> (element #1=w538:string, element #2=w536:string)  [unwired: 2 in]
          n199 = Build Array(w538) -> (w537:string[])
          n200 = Build Array(4 ("nData 2")) -> (w553:i32[])
          n201 = Build Array(5 ("nData 2")) -> (w548:i32[])
          n202 = call "CRYTree Manipulate Sub.vi"("sAction"="GetCellStringsbyColumn", "sData"=w537, "nData"=w553, "Tree in"=w535) -> ("sData Out"=w547:string[])  [unwired: 3 in, 4 out]
          n203 = call "CRYTree Manipulate Sub.vi"("sAction"="GetCellStringsbyColumn", "sData"=w537, "nData"=w548, "Tree in"=w535) -> ("sData Out"=w544:string[])  [unwired: 3 in, 4 out]
          n204 = Index Array(array=w547) -> (element=w546:string)  [unwired: 1 in]
          n205 = Index Array(array=w544) -> (element=w545:string)  [unwired: 1 in]
          n206 = Decimal String To Number(string=w546) -> (number=w540:i32)  [unwired: 2 in, 1 out]
          n207 = Decimal String To Number(string=w545) -> (number=w539:i32)  [unwired: 2 in, 1 out]
          n208 = call "CRYFind Insert Locaction in Tree.vi"("Index in Step"=w539, "Index in Tree"=w540, "ParentTag In"=w536, "Tree in"=w535) -> ("ChildIndex"=w541:i32, "ParentTag Out"=w542:string)  [unwired: 5 in, 1 out]
          n209 = Build Array(w542) -> (w555:string[])
          n210 = Build Array(w541) -> (w554:i32[])
        }
        frame "Drop" {
          # "Drop"
          n211 = Index Array(array=w559) -> (element #1=w563:string, element #2=w561:string)  [unwired: 2 in]
          n212 = Array Subset(array=w559, index=2) -> (w556:string[])  [unwired: 1 in]
          n213 = Build Array(w563) -> (w562:string[])
          n214 = Build Array(4 ("nData 2")) -> (w577:i32[])
          n215 = Build Array(5 ("nData 2")) -> (w572:i32[])
          n216 = call "CRYTree Manipulate Sub.vi"("sAction"="GetCellStringsbyColumn", "sData"=w562, "nData"=w577, "Tree in"=w560) -> ("sData Out"=w571:string[])  [unwired: 3 in, 4 out]
          n217 = call "CRYTree Manipulate Sub.vi"("sAction"="GetCellStringsbyColumn", "sData"=w562, "nData"=w572, "Tree in"=w560) -> ("sData Out"=w568:string[])  [unwired: 3 in, 4 out]
          n218 = Index Array(array=w571) -> (element=w570:string)  [unwired: 1 in]
          n219 = Index Array(array=w568) -> (element=w569:string)  [unwired: 1 in]
          n220 = Decimal String To Number(string=w570) -> (number=w565:i32)  [unwired: 2 in, 1 out]
          n221 = Decimal String To Number(string=w569) -> (number=w564:i32)  [unwired: 2 in, 1 out]
          n222 = call "CRYFind Insert Locaction in Tree.vi"("sData In"=w556, "sAction"="Drop", "Index in Step"=w564, "Index in Tree"=w565, "ParentTag In"=w561, "Tree in"=w560) -> ("ChildIndex"=w566:i32, "ParentTag Out"=w567:string)  [unwired: 3 in, 1 out]
          n223 = Build Array(w567) -> (w579:string[])
          n224 = Build Array(w566) -> (w578:i32[])
        }
        frame "Step" {
          n225 = global read "CRYCurve Library Global.vi" "CurveLib Info"() -> (w585:T3)
          n226 = Index Array(array=w589) -> (element #1=w581:i32, element #2=w582:i32)  [unwired: 2 in]
          n227 = Unbundle By Name(w585) -> ("GroupingState"=w586:string)
          n228 = case shown="\"Grouping by Category\"" w586 {
            tunnel: ["" w597 w634] -> w584
            tunnel: w583 -> [_ w596 w633]
            tunnel: w581 -> [_ w602 w631]
            tunnel: [_ w594 w628] -> w580
            frame "Grouping Off", Default {
            }
            frame "Grouping by Step" {
              n229 = Build Array("") -> (w605:string[])
              n230 = call "CRYTree Manipulate Sub.vi"("sAction"="GetTags", "sData"=w605, "sOption"="Childs", "Tree in"=w596) -> ("sData Out"=w599:string[], "Tree Out"=w595:refnum<vi>)  [unwired: 3 in, 3 out]
              n231 = for {
                tunnel: w599 -> [w621] mode=indexing
                shift-right: [w623] -> w600
                shift-left: w595 -> [w622]
                tunnel: w602 -> [w617]
                tunnel: [w614] -> w601
                tunnel: [w613] -> w598
                shift-right: [w612] -> w594
                shift-left: errorcluster {"status"=FALSE, "code"=0, "source"=""} ("error out") -> [w611]
                i -> [w613]
                stop <- w614 stop-if-true
                n232 = Build Array(w621) -> (w624:string[])
                n233 = property class="Tree"(reference=w622, error in=w611, "Active Item Tag"=w621, "ActiveColNum"=4 ("Active Cell:Active Column Number")) -> (error out=w612:errorcluster, "Cell String"=w619:string)  [unwired: 1 out]
                n234 = call "CRYTree Manipulate Sub.vi"("sAction"="CheckGroup", "sData"=w624, "sOption"="byTag", "Tree in"=w622) -> ("Tree Out"=w623:refnum<vi>, "bCategory"=w615:bool)  [unwired: 3 in, 3 out]
                n235 = Decimal String To Number(string=w619) -> (number=w618:i32)  [unwired: 2 in, 1 out]
                n236 = Equal?(x=w618, y=w617) -> (x = y?=w616:bool)
                n237 = And(x=w615, y=w616) -> (x .and. y?=w614:bool)
              }
              n238 = case shown="True" w601 {
                tunnel: w600 -> [_ _]
                tunnel: w599 -> [_ w610]
                tunnel: w598 -> [_ w609]
                tunnel: ["" w608] -> w597
                frame False {
                }
                frame True {
                  n239 = Index Array(array=w610, index=w609) -> (element=w608:string)
                }
              }
            }
            frame "Grouping by Category" {
              n240 = call "CRYGet Group Category.vi"("sOption"="VisibleIndex", "nData"=w631) -> ("sCategory"=w630:string)  [unwired: 9 in]
              n241 = Build Array("") -> (w641:string[])
              n242 = call "CRYTree Manipulate Sub.vi"("sAction"="GetTags", "sData"=w641, "sOption"="Childs", "Tree in"=w633) -> ("sData Out"=w636:string[], "Tree Out"=w632:refnum<vi>)  [unwired: 3 in, 3 out]
              n243 = for {
                tunnel: w636 -> [w650] mode=indexing
                shift-right: [w658] -> w637
                shift-left: w632 -> [w651]
                tunnel: [w655] -> w638
                tunnel: [w654] -> w635
                tunnel: w630 -> [w653]
                shift-right: [w648] -> w628
                shift-left: errorcluster {"status"=FALSE, "code"=0, "source"=""} ("error out") -> [w647]
                i -> [w654]
                stop <- w655 stop-if-true
                n244 = Build Array(w650) -> (w659:string[])
                n245 = property class="Tree"(reference=w651, error in=w647, "Active Item Tag"=w650, "ActiveColNum"=4 ("Active Cell:Active Column Number")) -> (error out=w648:errorcluster, "Cell String"=w649:string)  [unwired: 1 out]
                n246 = call "CRYTree Manipulate Sub.vi"("sAction"="CheckGroup", "sData"=w659, "sOption"="byTag", "Tree in"=w651) -> ("Tree Out"=w658:refnum<vi>, "bCategory"=w656:bool)  [unwired: 3 in, 3 out]
                n247 = Equal?(x=w649, y=w653) -> (x = y?=w657:bool)
                n248 = And(x=w656, y=w657) -> (x .and. y?=w655:bool)
              }
              n249 = case shown="True" w638 {
                tunnel: w637 -> [_ _]
                tunnel: w636 -> [_ w646]
                tunnel: w635 -> [_ w645]
                tunnel: ["" w644] -> w634
                frame False {
                }
                frame True {
                  n250 = Index Array(array=w646, index=w645) -> (element=w644:string)
                }
              }
            }
          }
          n251 = call "CRYFind Insert Locaction in Tree.vi"("Index in Step"=w582, "Index in Tree"=w581, "ParentTag In"=w584, "Tree in"=w583) -> ("ChildIndex"=w587:i32, "ParentTag Out"=w588:string)  [unwired: 5 in, 1 out]
          n252 = Build Array(w588) -> (w591:string[])
          n253 = Build Array(w587) -> (w590:i32[])
        }
        frame "StepDataGroup" {
          # "CRYGroup Manipulate.vi\\MakeGroup"
          n254 = Index Array(array=w668) -> (element=w665:i32)  [unwired: 1 in]
          n255 = global read "CRYCurve Library Global.vi" "CurveLib Info"() -> (w666:T3)
          n256 = Unbundle By Name(w666) -> ("GroupingState"=w667:string)
          n257 = case shown="\"Grouping by Category\"" w667 {
            tunnel: w663 -> [w672 w702]
            tunnel: w665 -> [w683 w704]
            tunnel: [w679 w703] -> w664
            tunnel: [w671 _] -> w662
            frame "Grouping by Step", Default {
              n258 = Build Array("") -> (w677:string[])
              n259 = call "CRYTree Manipulate Sub.vi"("sAction"="GetTags", "sData"=w677, "sOption"="Childs", "Tree in"=w672) -> ("sData Out"=w674:string[], "Tree Out"=w673:refnum<vi>)  [unwired: 3 in, 3 out]
              n260 = for {
                tunnel: w674 -> [w694] mode=indexing
                tunnel: w683 -> [w690]
                tunnel: [w687] -> w681
                tunnel: w673 -> [w695]
                tunnel: [w686] -> w682
                shift-right: [w685] -> w671
                shift-left: errorcluster {"status"=FALSE, "code"=0, "source"=""} ("error out") -> [w684]
                i -> [w687]
                stop <- w686 stop-if-true
                n261 = Build Array(w694) -> (w696:string[])
                n262 = property class="Tree"(reference=w695, error in=w684, "Active Item Tag"=w694, "ActiveColNum"=4 ("Active Cell:Active Column Number")) -> (error out=w685:errorcluster, "Cell String"=w692:string)  [unwired: 1 out]
                n263 = call "CRYTree Manipulate Sub.vi"("sAction"="CheckGroup", "sData"=w696, "sOption"="byTag", "Tree in"=w695) -> ("bCategory"=w688:bool)  [unwired: 3 in, 4 out]
                n264 = Decimal String To Number(string=w692) -> (number=w691:i32)  [unwired: 2 in, 1 out]
                n265 = Greater Or Equal?(x=w691, y=w690) -> (x >= y?=w689:bool)
                n266 = And(x=w688, y=w689) -> (x .and. y?=w686:bool)
              }
              n267 = Increment(x=w681) -> (x+1=w680:i32)
              n268 = Select(t=w681, s=w682, f=w680) -> (s? t:f=w679:i32)
            }
            frame "Grouping by Category" {
              n269 = call "CRYGet Group Category.vi"("sOption"="VisibleIndex", "nData"=w704) -> ("sCategory"=w701:string)  [unwired: 9 in]
              n270 = Build Array(w701) -> (w700:string[])
              n271 = call "CRYFind Insert Locaction in Tree Sub.vi"("sData In"=w700, "Tree In"=w702) -> ("ChildIndex"=w703:i32)  [unwired: 7 in, 2 out]
            }
          }
          n272 = Build Array(w664) -> (w669:i32[])
        }
        frame "UnGroup", Default {
          n273 = Index Array(array=w716) -> (element=w715:i32)  [unwired: 1 in]
          n274 = property on="Property Node" class="Tree"(reference=w713, "Active Item Row Number"=w715) -> (reference out=w718:refnum<vi>, error out=w717:errorcluster, "Active Item Tag"=w714:string)  [unwired: 1 in]
          n275 = invoke class="Tree" method="Navigate Tree.Get Parent"(reference=w718, error in=w717, "tag"=w714) -> (reference out=w710:refnum<vi>, error out=w706:errorcluster, "Navigate Tree:Get Parent"=w708:string)  [unwired: 1 in, 1 out]
          n276 = Empty String/Path?(string/path=w708) -> (empty?=w707:bool)
          n277 = case shown="False" w707 {
            tunnel: w710 -> [w723 _]
            tunnel: [w722 0 ("Active Item Row Number")] -> w709
            tunnel: w708 -> [w721 _]
            tunnel: w706 -> [w720 w724]
            tunnel: [w719 w724] -> w705
            frame False {
              n278 = property on="Property Node" class="Tree"(reference=w723, error in=w720, "Active Item Tag"=w721) -> (error out=w719:errorcluster, "Active Item Row Number"=w722:i32)  [unwired: 1 out]
            }
            frame True {
              # "Root"
            }
          }
          n279 = Build Array(w708) -> (w712:string[])
          n280 = Build Array(w709) -> (w711:i32[])
        }
      }
      n281 = local write "sData Out"(w371) -> ()
      n282 = local write "nData Out"(w370) -> ()
    }
    frame "GetTagsbyTreeNo" {
      n283 = property class="Tree"(reference=w735) -> (reference out=w733:refnum<vi>, error out=w727:errorcluster, "All Tags"=w734:string[])  [unwired: 1 in]
      n284 = Index Array(array=w732) -> (element=w731:i32)  [unwired: 1 in]
      n285 = Array Size(array=w734) -> (size(s)=w728:i32)
      n286 = for {
        N: w728 -> [_]
        tunnel: w733 -> [w753]
        tunnel: w731 -> [w750]
        shift-right: [w738] -> w729
        shift-left: string[] [] -> [w739]
        shift-right: [w736] -> w726
        shift-left: w727 -> [w737]
        i -> [w747]
        n287 = property class="Tree"(reference=w753, error in=w737, "Active Item Row Number"=w747, "ActiveColNum"=4 ("Active Cell:Active Column Number")) -> (reference out=w748:refnum<vi>, error out=w736:errorcluster, "Active Item Tag"=w740:string, "Cell String"=w752:string)
        n288 = Build Array(w747) -> (w746:i32[])
        n289 = Decimal String To Number(string=w752) -> (number=w751:i32)  [unwired: 2 in, 1 out]
        n290 = call "CRYTree Manipulate Sub.vi"("sAction"="CheckGroup", "nData"=w746, "Tree in"=w748) -> ("bData out"=w745:bool, "Tree Out"=w742:refnum<vi>)  [unwired: 4 in, 3 out]
        n291 = Equal?(x=w751, y=w750) -> (x = y?=w744:bool)
        n292 = Compound Arithmetic op=AND(invert w745, w744) -> (w743:bool)
        n293 = case shown="True" w743 {
          tunnel: w742 -> [_ _]
          tunnel: w740 -> [_ w756]
          tunnel: w739 -> [w754 w757]
          tunnel: [w754 w755] -> w738
          frame False {
          }
          frame True {
            n294 = Build Array (concatenate)(w757, w756) -> (w755:string[])
          }
        }
      }
      n295 = local write "sData Out"(w729) -> ()
    }
    frame "SetTreeNobyTags" {
      n296 = Index Array(array=w763) -> (element=w762:i32)  [unwired: 1 in]
      n297 = for {
        tunnel: w761 -> [w770]
        tunnel: w762 -> [w768]
        tunnel: w760 -> [w766] mode=indexing
        shift-right: [w765] -> w759
        shift-left: errorcluster {"status"=FALSE, "code"=0, "source"=""} ("error out") -> [w764]
        n298 = Number To Decimal String(number=w768) -> (decimal integer string=w767:string)  [unwired: 1 in]
        n299 = property class="Tree"(reference=w770, error in=w764, "Active Item Tag"=w766, "ActiveColNum"=4 ("Active Cell:Active Column Number"), "Cell String"=w767) -> (error out=w765:errorcluster)  [unwired: 1 out]
      }
    }
  }
  n300 = call "CRYCurve Library Error Message.vi"("sAction"="Curve", "sOption"="None", "error IO"=w1) -> ()  [unwired: 9 in]
  "Tree Out" <- "Tree in"
